vi "Master Setup Check Which Event Occured.vi"(5 "CtlRef":refnum<vi>, 7 "NewVal":bool) -> (0 "File Operations":T2, 2 "Event Occurred":T1, 3 "Sequence":string[](array[string]))   [LabVIEW 2017]
uses:
  Setup File Operations/File Operation with History.ctl
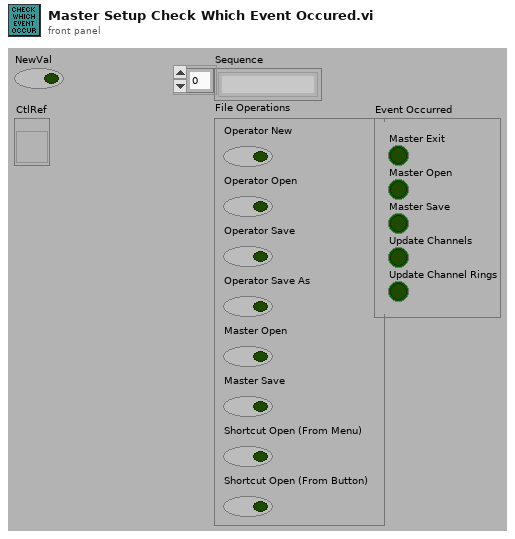
[diagram p1: front panel]
types:
  T1 = cluster{"Master Exit":bool, "Master Open":bool, "Master Save":bool, "Update Channels":bool, "Update Channel Rings":bool}
  T2 = typedef "File Operation with History.ctl" = cluster{"Operator New":bool, "Operator Open":bool, "Operator Save":bool, "Operator Save As":bool, "Master Open":bool, "Master Save":bool, "Shortcut Open (From Menu)":bool, "Shortcut Open (From Button)":bool}
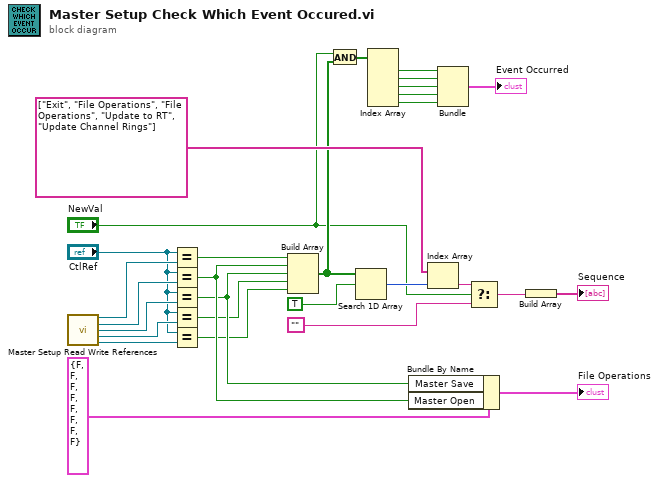
[diagram p0: block diagram]
diagram:
  n1 = call "Master Setup Read Write References.vi"() -> ("Master Exited (out)"=w18:refnum<vi>, "Master Open (out)"=w20:refnum<vi>, "Master Save (out)"=w21:refnum<vi>, "Update Channels (out)"=w23:refnum<vi>, "Update Channel Rings (out)"=w22:refnum<vi>)  [unwired: 10 in, 1 out]
  n2 = Equal?(x="CtlRef", y=w18) -> (x = y?=w14:bool)
  n3 = Equal?(x="CtlRef", y=w20) -> (x = y?=w13:bool)
  n4 = Equal?(x="CtlRef", y=w21) -> (x = y?=w12:bool)
  n5 = Equal?(x="CtlRef", y=w23) -> (x = y?=w11:bool)
  n6 = Equal?(x="CtlRef", y=w22) -> (x = y?=w10:bool)
  n7 = Build Array(w14, w13, w12, w11, w10) -> (w3:bool[])
  n8 = And(x="NewVal", y=w3) -> (x .and. y?=w1:bool[])
  n9 = Search 1D Array(1D array=w3, element=TRUE) -> (index of element=w25:i32)  [unwired: 1 in]
  n10 = Index Array(array=w1) -> (element #1=w8:bool, element #2=w7:bool, element #3=w6:bool, element #4=w5:bool, element #5=w4:bool)  [unwired: 5 in]
  n11 = Bundle By Name(cluster=T2 {"Operator New"=FALSE, "Operator Open"=FALSE, "Operator Save"=FALSE, "Operator Save As"=FALSE, "Master Open"=FALSE, "Master Save"=FALSE, "Shortcut Open (From Menu)"=FALSE, "Shortcut Open (From Button)"=FALSE} ("File Operations"), "Master Save"=w12, "Master Open"=w13) -> (→"File Operations":T2)
  n12 = Index Array(array=string[] ["Exit", "File Operations", "File Operations", "Update to RT", "Update Channel Rings"], index=w25) -> (element=w26:string)
  n13 = Bundle(w8, w7, w6, w5, w4) -> (→"Event Occurred":cluster{bool, bool, bool, bool, bool})  [unwired: 1 in]
  n14 = Select(t=w26, s="NewVal", f="") -> (s? t:f=w28:string)
  n15 = Build Array(w28) -> (→"Sequence":string[])
